vi "Write Harmonics.vi"(8 "error in (no error)":errorcluster, 10 "Harmonics":i8[](array[numeric]), 11 "Harmonics_Relative_Power in":refnum<class "Harmonics_Relative_Power.lvclass">=refnum) -> (0 "error out":errorcluster, 3 "Harmonics_Relative_Power out":refnum<class "Harmonics_Relative_Power.lvclass">)   [LabVIEW 2016, in "SeqAuto Evaluations.lvlib" / "Harmonics_Relative_Power.lvclass"]
uses:
  Harmonics_Relative_Power.lvclass
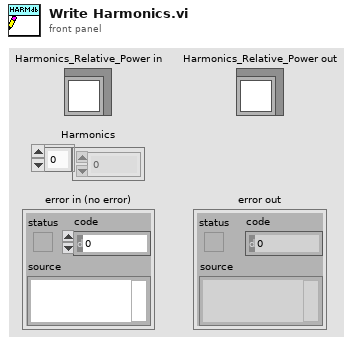
[diagram p1: front panel]
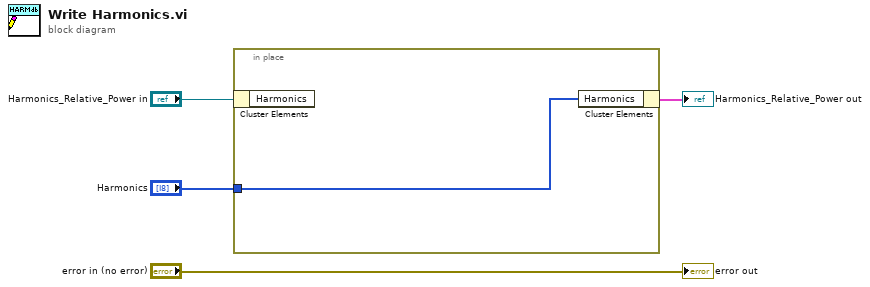
[diagram p0: block diagram]
diagram:
  n1 = in-place {
    in-place-border: "Harmonics" -> [w5]
    n2 = in-place-cluster #1("Harmonics_Relative_Power in") -> ()  [unwired: 1 out]
    n3 = in-place-cluster #1("Harmonics"=w5) -> (→"Harmonics_Relative_Power out":cluster{})
  }
  "error out" <- "error in (no error)"
